vi "Set Property.vi"(8 "error in (no error)":errorcluster, 9 "Value":dbl, 10 "Property":string, 11 "AM in":refnum<class "AM.lvclass">) -> (0 "error out":errorcluster, 3 "AM out":refnum<class "AM.lvclass">)   [LabVIEW 2015, in "AM.lvclass"]
uses:
  AM.lvclass
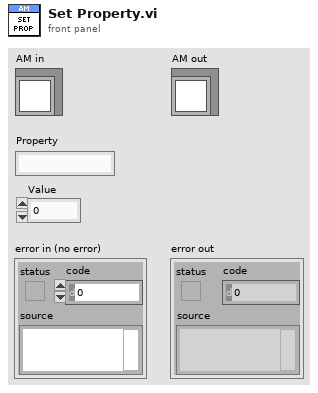
[diagram p1: front panel]
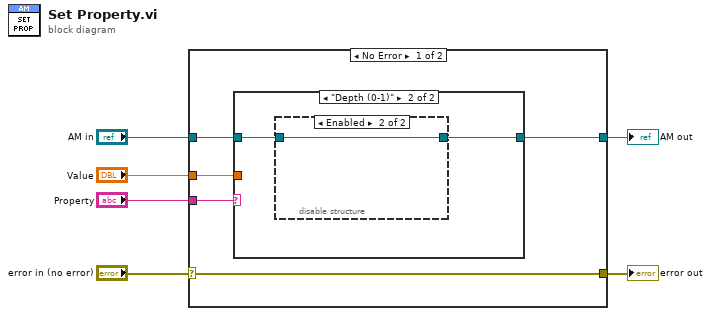
[diagram p0: block diagram]
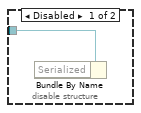
[diagram p3: hidden frame]
diagram:
  n1 = case shown="No Error" "error in (no error)" {
    selector: "error in (no error)" -> [w11 w18]
    tunnel: [w11 w18] -> w5
    tunnel: [w7 w17] -> w3
    tunnel: "AM in" -> [w10 w17]
    tunnel: "Property" -> [w9 _]
    tunnel: "Value" -> [w8 _]
    frame No Error {
      n2 = case shown="\"Depth (0-1)\"" w9 {
        tunnel: w10 -> [w12 w14]
        tunnel: w8 -> [_ _]
        tunnel: [w12 w13] -> w7
        frame "", Default {
        }
        frame "Depth (0-1)" {
          n3 = disable-structure shown="Enabled" {
            disable-tunnel: w14 -> [w15 w16]
            disable-tunnel: [_ w16] -> w13
            frame Disabled {
              n4 = Bundle By Name(cluster=w15) -> ()  [unwired: 1 in, 1 out]
            }
            frame Enabled {
            }
          }
        }
      }
    }
    frame Error {
    }
  }
  "error out" <- w5
  "AM out" <- w3
